vi "Config Element.vi"(11 "Seq Element in":refnum<class "Seq Element.lvclass">) -> (2 "Config Element":refnum<class "Config Element.lvclass">, 3 "Seq Element out":refnum<class "Seq Element.lvclass">)   [LabVIEW 2020, in "Seq Element.lvclass"]
uses:
  Seq Element.lvclass
  lv-cdm/CDM-Config/Config Element/Config Element.lvclass
  Seq Element.lvclass/Seq Element.ctl
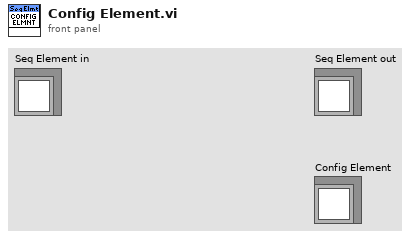
[diagram p1: front panel]
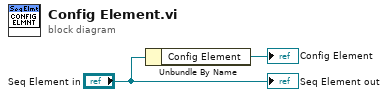
[diagram p0: block diagram]
diagram:
  n1 = Unbundle By Name("Seq Element in") -> ("Config Element"=→"Config Element":refnum<class "Config Element.lvclass">)
  "Seq Element out" <- "Seq Element in"
